vi "Training_Status.vi"() -> ()   [LabVIEW 2020]
panel:
  out "Training":bool
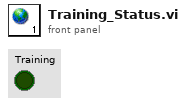
[diagram p1: front panel]
diagram:
